vi "PE Get Grating Wavelength Range.vi"(8 "error in (no error)":errorcluster, 10 "gratingIndex":i32, 11 "peHandle":u32) -> (0 "error out":errorcluster, 2 "maximum":dbl, 3 "minimum":dbl)   [LabVIEW 2017, in "PE_Filter_SDK.lvlib"]
doc: "PEFILTERSDK_API PE_STATUS PE_GetGratingWavelengthRange(CPE_HANDLE peHandle, int gratingIndex, double* minimum, double* maximum);"
uses:
  PE_Filter_SDK.lvlib
  PE_Filter_SDK.dll
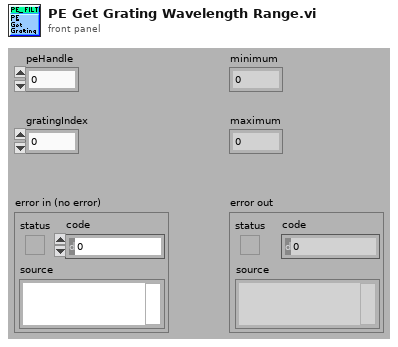
[diagram p1: front panel]
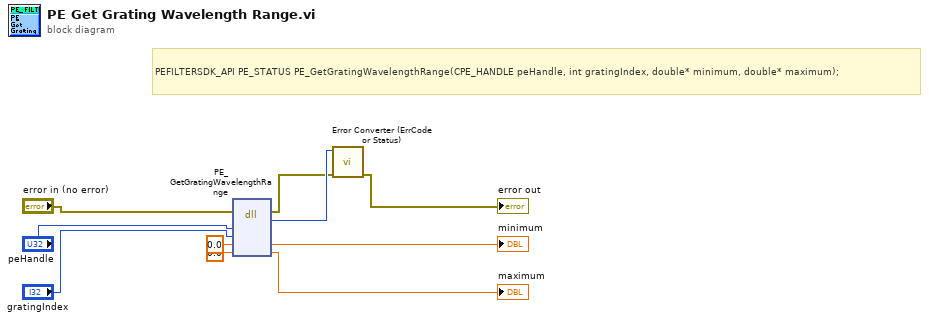
[diagram p0: block diagram]
diagram:
  # "PEFILTERSDK_API PE_STATUS PE_GetGratingWavelengthRange(CPE_HANDLE peHandle, int gratingIndex, double* minimum, double* maximum);"
  n1 = dll-call lib="D:/working_directory/SDK LLTF/trunk_commit/examples/PE_Filter_SDK/PE_Filter_SDK.*" fn="PE_GetGratingWavelengthRange"(error in="error in (no error)", "peHandle"="peHandle", "gratingIndex"="gratingIndex", "minimum"=0.0, "maximum"=0.0) -> (error out=w2:errorcluster, w3:u32, "minimum"=→"minimum":dbl, "maximum"=→"maximum":dbl)  [unwired: 4 in, 1 out]
  n2 = call "Error Converter (ErrCode or Status).vi"("error in (no error)"=w2, "error code"=w3) -> ("error out"=→"error out":errorcluster)  [unwired: 9 in]
